vi "Advanced DC-RMS Measurement.vi"() -> ()   [LabVIEW 2020]
doc: "Demonstrates how to compute the DC and RMS value of a signal."
uses:
  <vilib>/measure/madcrms.llb/Averaged DC-RMS for 1 Chan.vi
  <vilib>/measure/NI_MAPro.lvlib
panel:
  in  "Averaging Window":u16(ring) items=["Rectangular (none)", "Hanning", "Low side lobe"]
  in  "Averaging Time":dbl=0.01
  in  "Averaging Type":u16(ring) items=["Linear", "Exponential"]
  in  "Stop":bool
  out "Measurement Results":waveform(dbl)[](graph)
  out "Test Signal":waveform(dbl)(graph)
  # "Overview: Demonstrates the use of the Averaged DC-RMS VI.\nRequirements: LabVIEW Full Development System\nInstructions:\n1. Run the VI. Observe the DC and RMS values obtained from the test signal.\n2. Click Stop to stop the VI."
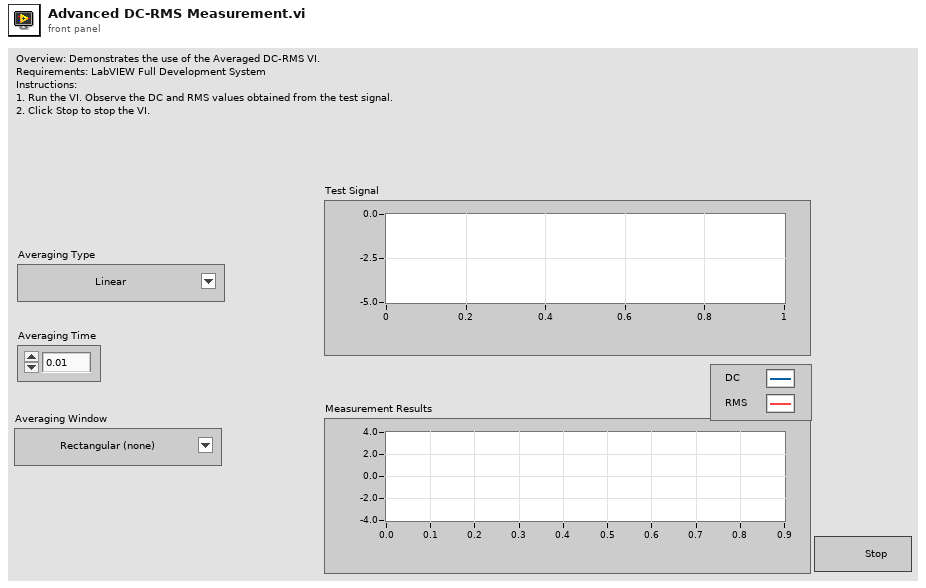
[diagram p1: front panel]
types:
  T1 = enum16{"Rectangular (none)", "Hanning", "Low side lobe"}
  T2 = cluster{"window for DC":enum16{"Rectangular (none)", "Hanning", "Low side lobe"}, "output function":enum16{"DC only", "RMS only", "DC and RMS"}, "window for RMS":enum16{"Rectangular (none)", "Hanning", "Low side lobe"}, "exp. time constant":dbl, "Ignore input start time":bool}
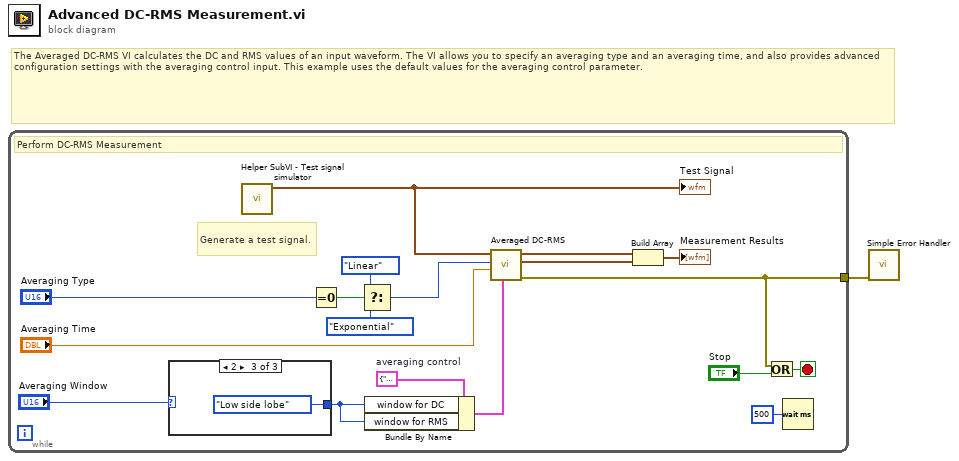
[diagram p0: block diagram]
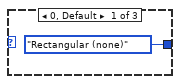
[diagram p2: hidden frame]
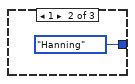
[diagram p3: hidden frame]
diagram:
  # "The Averaged DC-RMS VI calculates the DC and RMS values of an input waveform. The VI allows you to specify an averaging type and an averaging time, and also provides advanced configuration settings with the averaging control input. This example uses the default values for the averaging control parameter."
  n1 = while {
    tunnel: [w12] -> w1
    stop <- w13 stop-if-true
    w5 = T2 {"window for DC"=enum."Rectangular (none)", "output function"=enum."DC and RMS", "window for RMS"=enum."Rectangular (none)", "exp. time constant"=-1.0, "Ignore input start time"=FALSE}  # averaging control
    # "Generate a test signal."
    # "Perform DC-RMS Measurement"
    n2 = case shown="2" "Averaging Window" {
      tunnel: [T1."Rectangular (none)" ("window for DC") T1."Hanning" ("window for DC") T1."Low side lobe" ("window for DC")] -> w2
      frame 0, Default {
      }
      frame 1 {
      }
      frame 2 {
      }
    }
    n3 = call "Helper SubVI - Test signal simulator.vi"() -> ("Test Signal"=w14:waveform(dbl))  [unwired: 11 in]
    "Test Signal" <- w14
    n4 = Equal To 0?(x="Averaging Type") -> (x = 0?=w10:bool)
    n5 = Select(t=enum16{"Linear", "Exponential"}."Linear" ("averaging type"), s=w10, f=enum16{"Linear", "Exponential"}."Exponential" ("averaging type")) -> (s? t:f=w7:enum16{"Linear", "Exponential"})
    n6 = Bundle By Name(cluster=w5, "window for DC"=w2, "window for RMS"=w2) -> (w4:T2)
    n7 = call-poly <vilib>:"Averaged DC-RMS.vi"("averaging control"=w4, "averaging time"="Averaging Time", "averaging type"=w7, "signal in"=w14) -> ("error out"=w12:errorcluster, "RMS value waveform"=w15:waveform(dbl), "DC value waveform"=w16:waveform(dbl))  [unwired: 3 in, 2 out]
    n8 = Build Array(w16, w15) -> (→"Measurement Results":waveform(dbl)[])
    n9 = Or(x=w12, y="Stop") -> (x .or. y?=w13:bool)
    n10 = Wait (ms)(milliseconds to wait=u32 500) -> ()  [unwired: 1 out]
  }
  n11 = call <vilib>:"Simple Error Handler.vi"("error in (no error)"=w1) -> ()  [unwired: 4 in, 5 out]
